vi "Set Value of LabVIEW Array.vi"(8 "error in (no error)":errorcluster, 10 "LabVIEW Array":refnum<vi>, 11 "JSON Tree Array":variant) -> (0 "error out":errorcluster)   [LabVIEW 2014, in "i3-json.lvlib"]
doc: "This VI takes a JSON Node (all types besides JSON Object) and assigns the value to the LabVIEW Base Type of compatible reference.\n\nIf the LabVIEW base type is an array of boolean, numeric, or string this function will attempt to check if a JSON Array type will map"
uses:
  i3-json.lvlib
  Error Handling/Throw JSON Error Files/Throw JSON Error - Invalid Type Error.vi
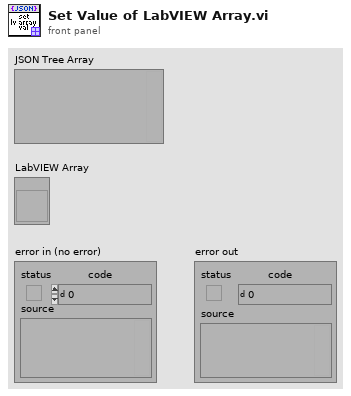
[diagram p1: front panel]
types:
  T1 = enum8{"Enabled", "Disabled", "Disabled and Grayed Out"}
  T2 = enum8{"Invalid Type", "Void", "I8", "I16", "I32", "I64", "U8", "U16", "U32", "U64", "Single Float", "Double Float", "Extended Float", "Single Complex", "Double Complex", "Extended Complex", "Enum U8", "Enum U16", "Enum U32", "Enum U64", "Single Float With Unit", "Double Float With Unit", "Extended Float With Unit", "Single Complex with Unit", "Double Complex with Unit", "Extended Complex with Unit", "Boolean", "String", "Path", "Picture", "Tag", "Array", "Cluster", "Variant", "LV Variant", "Waveform", "Timestamp", "Digital Waveform", "Digital Data", "ExpressData", "Refnum", "External Data", "VI", "Poly VI", "LabVIEW Class Instance", "Fixed Point"}
  T3 = typedef "i3-json.lvlib/JSON Type.ctl" = enum8{"JSON Compatible", "JSON Array", "JSON Object", "JSON Null", "Double", "String", "Boolean", "Unknown"}
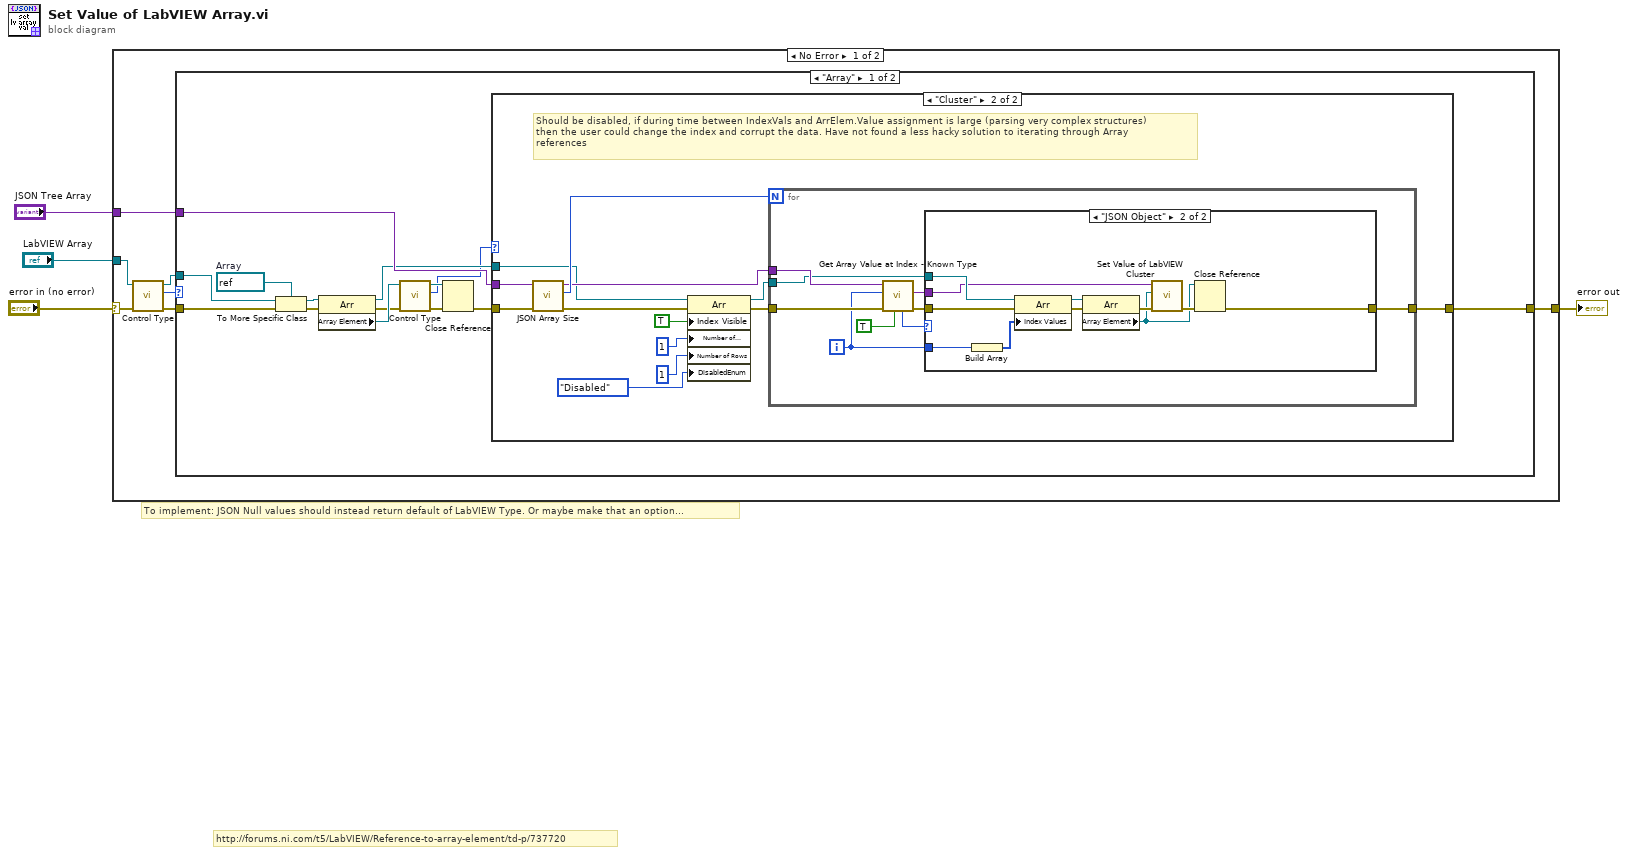
[diagram p0: block diagram]
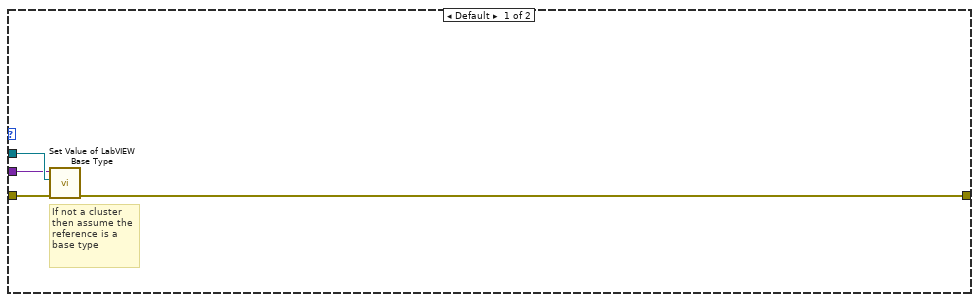
[diagram p2: hidden frame]
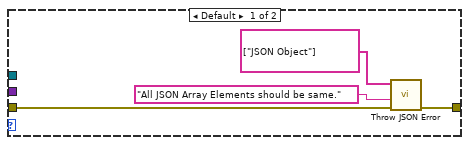
[diagram p3: hidden frame]
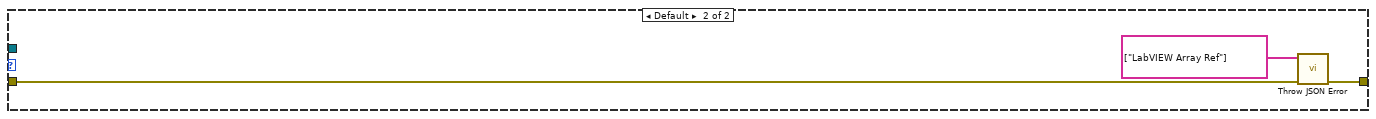
[diagram p4: hidden frame]
diagram:
  # "http://forums.ni.com/t5/LabVIEW/Reference-to-array-element/td-p/737720"
  # "To implement: JSON Null values should instead return default of LabVIEW Type. Or maybe make that an option..."
  n1 = case shown="No Error" "error in (no error)" {
    selector: "error in (no error)" -> [w9 w70]
    tunnel: "LabVIEW Array" -> [w7 _]
    tunnel: "JSON Tree Array" -> [w11 _]
    tunnel: [w10 w70] -> w1
    frame No Error {
      n2 = call "Control Type.vi"("error in (no error)"=w9, "Control in"=w7) -> ("error out"=w8:errorcluster, "Type"=w5:T2, "Control out"=w6:refnum<vi>)  [unwired: 7 in]
      n3 = case shown="\"Array\"" w5 {
        tunnel: w6 -> [w24 _]
        tunnel: w11 -> [w22 _]
        tunnel: w8 -> [w25 w67]
        tunnel: [w20 w68] -> w10
        frame "Array" {
          w21 = refnum<vi> refnum  # Array
          n4 = To More Specific Class(target class=w21, reference=w24, error in=w25) -> (specific class reference=w19:refnum<vi>, error out=w23:errorcluster)
          n5 = property class="Arr"(reference=w19, error in=w23) -> (reference out=w17:refnum<vi>, error out=w12:errorcluster, "Array Element"=w16:refnum<vi>)
          n6 = call "Control Type.vi"("error in (no error)"=w12, "Control in"=w16) -> ("error out"=w13:errorcluster, "Type"=w14:T2, "Control out"=w15:refnum<vi>)  [unwired: 7 in]
          n7 = Close Reference(reference=w15, error in (no error)=w13) -> (error out=w18:errorcluster)
          n8 = case shown="\"Cluster\"" w14 {
            tunnel: w18 -> [w29 w42]
            tunnel: w22 -> [w27 w41]
            tunnel: w17 -> [w28 w32]
            tunnel: [w26 w30] -> w20
            frame Default {
              # "If not a cluster then assume the reference is a base type"
              n9 = call "Set Value of LabVIEW Base Type.vi"("error in (no error)"=w29, "LabVIEW Base Type"=w28, "JSON Tree Node"=w27) -> ("error out"=w26:errorcluster)  [unwired: 8 in]
            }
            frame "Cluster" {
              # "Should be disabled, if during time between IndexVals and ArrElem.Value assignment is large (parsing very complex structures)\nthen the user could change the index and corrupt the data. Have not found a less hacky solution to iterating through Array\nreferences"
              n10 = call "JSON Array Size.vi"("error in (no error)"=w42, "JSON Tree In (JSON Array)"=w41) -> ("error out"=w34:errorcluster, "Array Size"=w40:i32, "JSON Tree Passthrough (JSON Array)"=w39:variant)  [unwired: 7 in]
              n11 = property class="Arr"(reference=w32, error in=w34, "Index Visible"=TRUE, "Number of Columns"=u32 1, "Number of Rows"=u32 1, "DisabledEnum"=T1."Disabled" ("Disabled")) -> (reference out=w31:refnum<vi>, error out=w33:errorcluster)
              n12 = for {
                N: w40 -> [_]
                tunnel: w39 -> [w50]
                tunnel: w33 -> [w51]
                tunnel: w31 -> [w45]
                tunnel: [w46] -> w30
                i -> [w44]
                n13 = call "Get Array Value at Index - Known Type.vi"("Get Value as JSON Tree? (F)"=TRUE, "error in (no error)"=w51, "Index"=w44, "JSON Tree In (JSON Array)"=w50) -> ("error out"=w48:errorcluster, "Value"=w47:variant, "JSON Type"=w49:T3)  [unwired: 2 in, 3 out]
                n14 = case shown="\"JSON Object\"" w49 {
                  tunnel: w48 -> [w53 w66]
                  tunnel: w47 -> [_ w59]
                  tunnel: [w52 w58] -> w46
                  tunnel: w45 -> [_ w63]
                  tunnel: w44 -> [_ w65]
                  frame Default {
                    n15 = call-poly "Throw JSON Error.vi"("error in (no error)"=w53, "additional info"="All JSON Array Elements should be same." ("source"), "Valid Types"=string[] ["JSON Object"]) -> ("error out"=w52:errorcluster)  [unwired: 8 in]
                  }
                  frame "JSON Object" {
                    n16 = Build Array(w65) -> (w64:i32[])
                    n17 = property class="Arr"(reference=w63, error in=w66, "Index Values"=w64) -> (reference out=w62:refnum<vi>, error out=w61:errorcluster)
                    n18 = property class="Arr"(reference=w62, error in=w61) -> (error out=w60:errorcluster, "Array Element"=w56:refnum<vi>)  [unwired: 1 out]
                    n19 = call "Set Value of LabVIEW Cluster.vi"("error in (no error)"=w60, "LabVIEW Cluster"=w56, "JSON Tree Object"=w59) -> ("error out"=w57:errorcluster)  [unwired: 8 in]
                    n20 = Close Reference(reference=w56, error in (no error)=w57) -> (error out=w58:errorcluster)
                  }
                }
              }
            }
          }
        }
        frame Default {
          n21 = call-poly "Throw JSON Error.vi"("error in (no error)"=w67, "Valid Types"=string[] ["LabVIEW Array Ref"]) -> ("error out"=w68:errorcluster)  [unwired: 9 in]
        }
      }
    }
    frame Error {
    }
  }
  "error out" <- w1
